vi "dfd_Group Delay_Add Band1.vi"(6 "grid length":dbl, 8 "weight (in)":dbl[](array[numeric]), 9 "d (in)":dbl[](array[numeric]), 10 "freq grid (in)":dbl[](array[numeric]), 11 "allpass band spec":T1[](array[typedef]) {"subband specs"."weight" format="%.2f"}) -> (0 "weight (out)":dbl[](array[numeric]), 1 "d (out)":dbl[](array[numeric]), 2 "freq grid (out)":dbl[](array[numeric]), 3 "allpass band spec (dup)":T1[](array[typedef]) {"subband specs"."weight" format="%.2f"})   [LabVIEW 2017, in "NI_DigFilter_Design.lvlib"]
uses:
  <vilib>/addons/Digital Filter Design/NI_DigFilter_Design.lvlib
  <vilib>/addons/Digital Filter Design/_GroupDelay.llb/dfd_Group Delay_Band Spec.ctl
  <vilib>/addons/Digital Filter Design/NI_DigFilterLicensed.lvlib
panel:
  # "freq"
  # "group delay"
  # "weight"
  # "freq"
  # "group delay"
  # "weight"
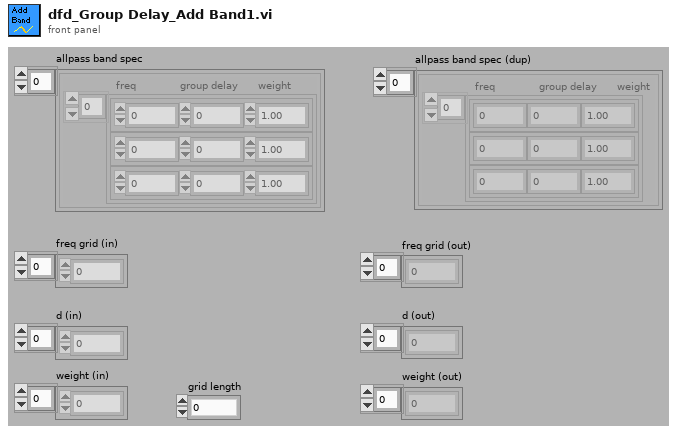
[diagram p1: front panel]
types:
  T1 = typedef "NI_DigFilterLicensed.lvlib/dfd_Group Delay_Band Spec.ctl" = cluster{"subband specs":cluster{"freq":dbl, "group delay":dbl, "weight":dbl}[]}
  T2 = cluster{"freq":dbl, "group delay":dbl, "weight":dbl}[]
  T3 = cluster{"freq":dbl, "group delay":dbl, "weight":dbl}
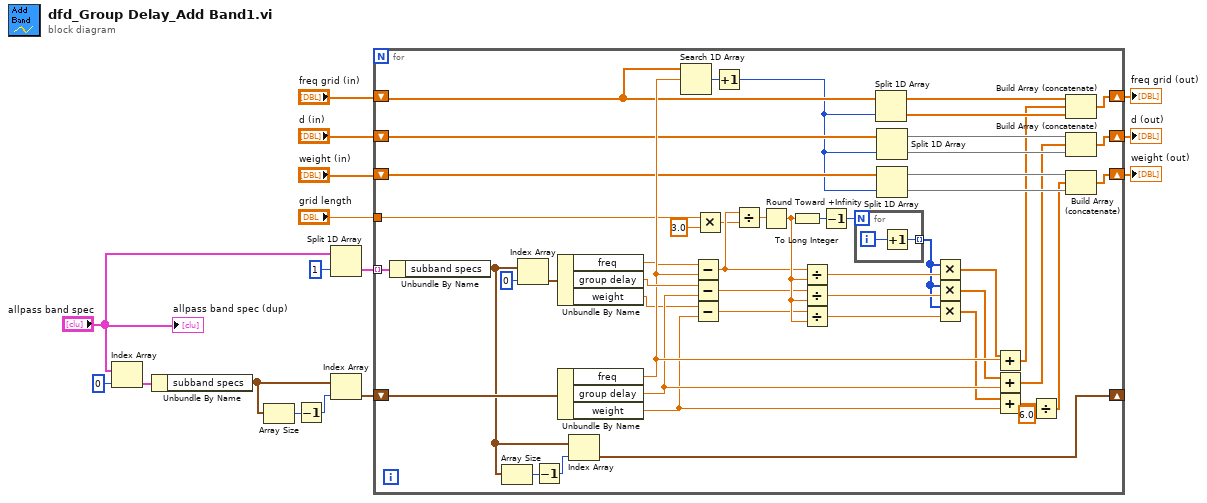
[diagram p0: block diagram]
diagram:
  n1 = Index Array(array="allpass band spec", index=0) -> (element=w9:T1)
  n2 = Unbundle By Name(w9) -> ("subband specs"=w14:T2)
  n3 = Array Size(array=w14) -> (size(s)=w15:i32)
  n4 = Decrement(x=w15) -> (x-1=w13:i32)
  n5 = Split 1D Array(array="allpass band spec", index=1) -> (second subarray=w11:T1[])  [unwired: 1 out]
  n6 = Index Array(array=w14, index=w13) -> (element=w12:T3)
  n7 = for {
    tunnel: w11 -> [w59] mode=indexing
    shift-right: [w55] -> _
    shift-left: w12 -> [w65]
    shift-right: [w49] -> w2
    shift-left: "weight (in)" -> [w52]
    shift-right: [w50] -> w3
    shift-left: "d (in)" -> [w53]
    shift-right: [w51] -> w4
    shift-left: "freq grid (in)" -> [w54]
    tunnel: "grid length" -> [w17]
    n8 = Unbundle By Name(w59) -> ("subband specs"=w56:T2)
    n9 = Array Size(array=w56) -> (size(s)=w58:i32)
    n10 = Index Array(array=w56, index=0) -> (element=w60:T3)
    n11 = Decrement(x=w58) -> (x-1=w57:i32)
    n12 = Unbundle By Name(w60) -> ("freq"=w47:dbl, "group delay"=w64:dbl, "weight"=w48:dbl)
    n13 = Unbundle By Name(w65) -> ("freq"=w63:dbl, "group delay"=w62:dbl, "weight"=w61:dbl)
    n14 = Index Array(array=w56, index=w57) -> (element=w55:T3)
    n15 = Search 1D Array(1D array=w54, element=w63) -> (index of element=w39:i32)  [unwired: 1 out]
    n16 = Subtract(x=w47, y=w63) -> (x-y=w44:dbl)
    n17 = Subtract(x=w64, y=w62) -> (x-y=w43:dbl)
    n18 = Subtract(x=w48, y=w61) -> (x-y=w42:dbl)
    n19 = Multiply(x=w17, y=3.0) -> (x*y=w29:dbl)
    n20 = Increment(x=w39) -> (x+1=w38:i32)
    n21 = Divide(x=w44, y=w29) -> (x/y=w46:dbl)
    n22 = Round Toward +Infinity(x=w46) -> (ceil(x): smallest int >= x=w45:dbl)
    n23 = To Long Integer(number=w45) -> (32bit integer=w41:i32)
    n24 = Divide(x=w44, y=w45) -> (x/y=w25:dbl)
    n25 = Divide(x=w43, y=w45) -> (x/y=w27:dbl)
    n26 = Divide(x=w42, y=w45) -> (x/y=w26:dbl)
    n27 = Decrement(x=w41) -> (x-1=w40:i32)
    n28 = for {
      N: w40 -> [_]
      tunnel: [w67] -> w24 mode=indexing
      i -> [w68]
      n29 = Increment(x=w68) -> (x+1=w67:i32)
    }
    n30 = Split 1D Array(array=w54, index=w38) -> (first subarray=w37:dbl[], second subarray=w36:dbl[])
    n31 = Split 1D Array(array=w53, index=w38) -> (first subarray=w35:dbl[], second subarray=w34:dbl[])
    n32 = Split 1D Array(array=w52, index=w38) -> (first subarray=w33:dbl[], second subarray=w32:dbl[])
    n33 = Multiply(x=w24, y=w25) -> (x*y=w20:dbl[])
    n34 = Multiply(x=w24, y=w27) -> (x*y=w19:dbl[])
    n35 = Multiply(x=w24, y=w26) -> (x*y=w18:dbl[])
    n36 = Add(x=w20, y=w63) -> (x+y=w21:dbl[])
    n37 = Add(x=w19, y=w62) -> (x+y=w22:dbl[])
    n38 = Add(x=w18, y=w61) -> (x+y=w23:dbl[])
    n39 = Divide(x=w23, y=6.0) -> (x/y=w31:dbl[])
    n40 = Build Array (concatenate)(w37, w21, w36) -> (w51:dbl[])
    n41 = Build Array (concatenate)(w35, w22, w34) -> (w50:dbl[])
    n42 = Build Array (concatenate)(w33, w31, w32) -> (w49:dbl[])
  }
  "weight (out)" <- w2
  "freq grid (out)" <- w4
  "d (out)" <- w3
  "allpass band spec (dup)" <- "allpass band spec"
